vi "Write inputs.vi"(5 "inputs":refnum<class "Terminal.lvclass">[](array[class]), 9 "Node in":refnum<class "Node.lvclass">) -> (3 "Node out":refnum<class "Node.lvclass">)   [LabVIEW 2014, in "Node.lvclass"]
uses:
  Node.lvclass
  Terminal/Terminal.lvclass
  Node.lvclass/Node.ctl
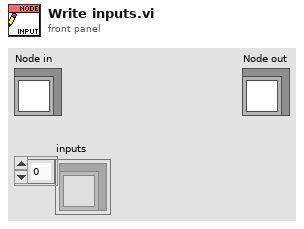
[diagram p1: front panel]
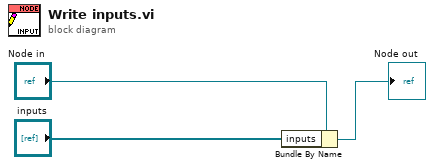
[diagram p0: block diagram]
diagram:
  n1 = Bundle By Name(cluster="Node in", "inputs"="inputs") -> (→"Node out":refnum<class "Node.lvclass">)
